vi "Format Indent.vi"(9 "Indent":i32, 11 "XML in":refnum<class "XML.lvclass">) -> (1 "Indent out":i32, 3 "XML out":refnum<class "XML.lvclass">, 4 "Indent XML":string)   [LabVIEW 2019, in "XML.lvlib" / "XML.lvclass"]
uses:
  <vilib>/gpm_packages/@cs/persistence/source/XML/XML.lvclass
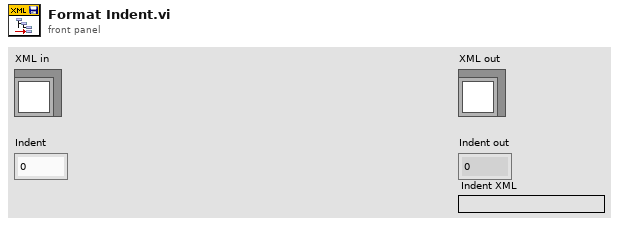
[diagram p1: front panel]
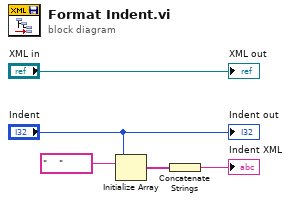
[diagram p0: block diagram]
diagram:
  n1 = Initialize Array("    ", "Indent") -> (w3:string[])
  n2 = Concatenate Strings(w3) -> (→"Indent XML":string)
  "XML out" <- "XML in"
  "Indent out" <- "Indent"
